vi "Wait for Configured Network.vi"(9 "must be directly reachable? (F)":bool, 10 "timeout in ms":i32=-1, 11 "hostname or URL in":string) -> (2 "network status for remote host":T1, 3 "hostname or URL out":string)   [LabVIEW 2020, in "NI_WFCN.lvlib"]
doc: "Waits until the system can contact the remote host."
uses:
  <vilib>/net/WFCN/NI_WFCN.lvlib
  <vilib>/net/WFCN/Network Status.ctl
  <vilib>/net/WFCN/Addressing/IPv4 Network Address/IPv4 Network Address.lvclass/IPv4 Network Address.ctl
  <vilib>/net/WFCN/Addressing/Generic Network Address/Generic Network Address.lvclass/Generic Network Address.ctl
  <vilib>/net/WFCN/Addressing/Hostname Network Address/Hostname Network Address.lvclass/Hostname Network Address.ctl
  <vilib>/net/WFCN/Get Default Timeout.vi
  <vilib>/net/WFCN/Addressing/Generic Network Address/Parse.vi
  <vilib>/net/WFCN/Interpret Network Status.vi
  <vilib>/net/WFCN/Addressing/Hostname Network Address/Create from string.vi
  <vilib>/net/WFCN/Utility/Is IPv4 address.vi
  <vilib>/net/WFCN/Addressing/IPv4 Network Address/Create from U32.vi
  <vilib>/net/WFCN/Addressing/Generic Network Address/Create for unparsable.vi
  <vilib>/net/WFCN/Utility/Is hostname mDNS.vi
  <vilib>/dlg_ctls.llb/Space Constant.vi
  <vilib>/net/WFCN/Addressing/IPv4 Network Address/IPv4 Network Address.lvclass
  e:/builds/penguin/labview/branches/2020/dev/dist/vi.lib/net/WFCN/Addressing/Generic Network Address/Generic Network Address.lvclass
  <vilib>/net/WFCN/Addressing/Hostname Network Address/Hostname Network Address.lvclass
  <vilib>/net/WFCN/Addressing/mDNS Hostname Network Address/mDNS Hostname Network Address.lvclass
  e:/builds/penguin/labview/branches/2020/dev/dist/vi.lib/net/WFCN/Addressing/Hostname Network Address/Hostname Network Address.lvclass
  <vilib>/Utility/error.llb/Error Cluster From Error Code.vi
  <vilib>/net/WFCN/Addressing/Generic Network Address/Select Best Address.vi
  <vilib>/UDC/API_Files/UDCCountUsage.vi
  <vilib>/net/WFCN/Addressing/Generic Network Address/Generic Network Address.lvclass
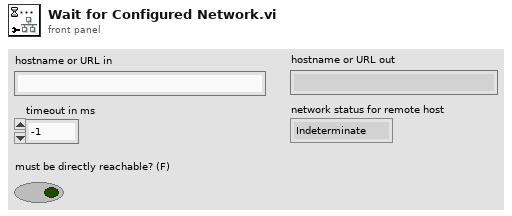
[diagram p1: front panel]
types:
  T1 = typedef "NI_WFCN.lvlib/Network Status.ctl" = enum16{"Indeterminate", "Configured", "Unconfigured"}
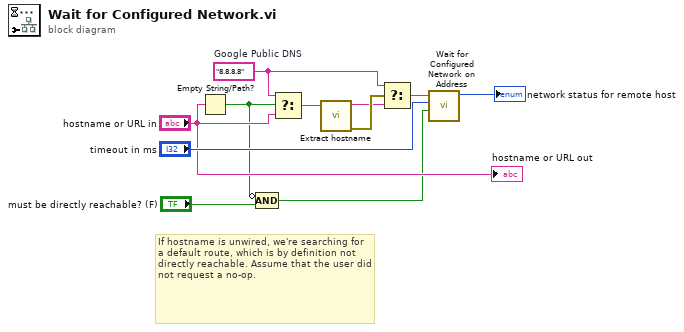
[diagram p0: block diagram]
diagram:
  w7 = "8.8.8.8"  # Google Public DNS
  # "If hostname is unwired, we're searching for a default route, which is by definition not directly reachable. Assume that the user did not request a no-op."
  n1 = Empty String/Path?(string/path="hostname or URL in") -> (empty?=w2:bool)
  n2 = Compound Arithmetic op=AND(invert w2, "must be directly reachable? (F)") -> (w1:bool)
  n3 = Select(t=w7, s=w2, f="hostname or URL in") -> (s? t:f=w9:string)
  n4 = call <vilib>:"Extract hostname.vi"("address or URI"=w9) -> ("error out"=w8:errorcluster, "hostname"=w6:string)  [unwired: 7 in]
  n5 = Select(t=w7, s=w8, f=w6) -> (s? t:f=w5:string)
  n6 = call <vilib>:"Wait for Configured Network on Address.vi"("must be directly reachable?"=w1, "timeout in ms"="timeout in ms", "address"=w5) -> ("network status for remote host"=→"network status for remote host":T1)  [unwired: 7 in, 1 out]
  "hostname or URL out" <- "hostname or URL in"
